vi "Set member data - output.vi"(8 "error in (no error)":errorcluster, 10 "rf on?":bool, 11 "Microwave.lvclass in":refnum<class "Microwave.lvclass">) -> (0 "error out":errorcluster, 3 "Microwave.lvclass out":refnum<class "Microwave.lvclass">)   [LabVIEW 2009, in "Microwave.lvclass"]
uses:
  Microwave.lvclass
  Microwave.lvclass/Microwave.ctl
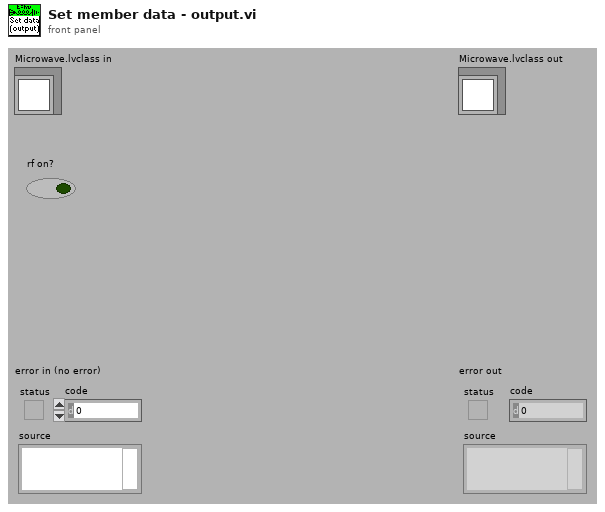
[diagram p1: front panel]
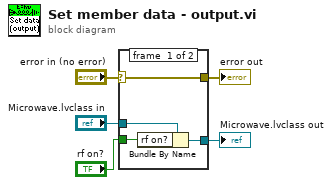
[diagram p0: block diagram]
diagram:
  n1 = case shown="No Error" "error in (no error)" {
    selector: "error in (no error)" -> [w9 w10]
    tunnel: [w9 w10] -> w4
    tunnel: [w6 w11] -> w2
    tunnel: "Microwave.lvclass in" -> [w7 w11]
    tunnel: "rf on?" -> [w8 _]
    frame #0 {
      n2 = Bundle By Name(cluster=w7, "rf on?"=w8) -> (w6:refnum<class "Microwave.lvclass">)
    }
    frame #1 {
    }
  }
  "error out" <- w4
  "Microwave.lvclass out" <- w2
